vi "PQexecute.vi"(8 "error in":errorcluster, 10 "SQL querry":string, 11 "conn":u64) -> (0 "error out":errorcluster, 3 "conn_out":u64)   [LabVIEW 2019, in "libpqutility64.lvlib"]
uses:
  libpqutility64.lvlib
  libpqlv64/libpqlv64.lvlib
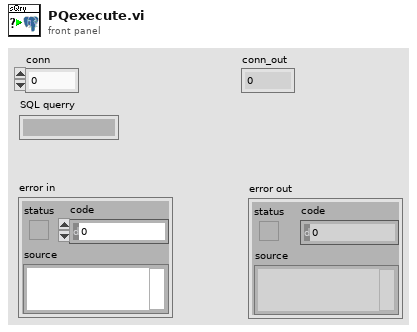
[diagram p1: front panel]
types:
  T1 = enum32{"PGRES_EMPTY_QUERY", "PGRES_COMMAND_OK", "PGRES_TUPLES_OK", "PGRES_COPY_OUT", "PGRES_COPY_IN", "PGRES_BAD_RESPONSE", "PGRES_NONFATAL_ERROR", "PGRES_FATAL_ERROR"}
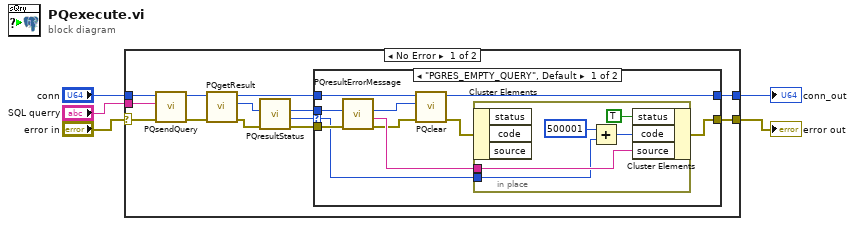
[diagram p0: block diagram]
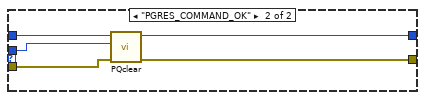
[diagram p2: hidden frame]
diagram:
  n1 = case shown="No Error" "error in" {
    selector: "error in" -> [w14 w39]
    tunnel: "conn" -> [w13 w40]
    tunnel: [w6 w40] -> w2
    tunnel: [w16 w39] -> w1
    tunnel: "SQL querry" -> [w15 _]
    frame No Error {
      n2 = call "PQsendQuery.vi"("error in (no error)"=w14, "query"=w15, "conn"=w13) -> ("error out"=w18:errorcluster, "conn_out"=w12:u64)  [unwired: 6 in, 1 out]
      n3 = call "PQgetResult.vi"("error in (no error)"=w18, "conn"=w12) -> ("error out"=w17:errorcluster, "PGresult"=w11:u64, "conn_out"=w7:u64)  [unwired: 7 in]
      n4 = call "PQresultStatus.vi"("error in (no error)"=w17, "res"=w11) -> ("error out"=w8:errorcluster, "PQresultStatus"=w10:T1, "res out"=w9:u64)  [unwired: 7 in]
      n5 = case shown="\"PGRES_EMPTY_QUERY\", Default" w10 {
        selector: w10 -> [w26 _]
        tunnel: [w25 w36] -> w16
        tunnel: w9 -> [w24 w38]
        tunnel: w8 -> [w28 w37]
        tunnel: w7 -> [w23 w35]
        tunnel: [w20 w34] -> w6
        frame "PGRES_EMPTY_QUERY", Default {
          n6 = call "PQresultErrorMessage.vi"("error in (no error)"=w28, "res"=w24) -> ("error out"=w22:errorcluster, "PQresultErrorMessage"=w27:string, "res out"=w21:u64)  [unwired: 7 in]
          n7 = call "PQclear.vi"("error in"=w22, "res"=w21, "conn"=w23) -> ("error out"=w19:errorcluster, "conn_out"=w20:u64)  [unwired: 7 in]
          n8 = in-place {
            in-place-border: w27 -> [w33]
            in-place-border: w26 -> [w30]
            n9 = in-place-cluster #1(w19) -> ()  [unwired: 3 out]
            n10 = Add(x=u32 500001, y=w30) -> (x+y=w29:u32)
            n11 = in-place-cluster #1("status"=TRUE, "code"=w29, "source"=w33) -> (w25:errorcluster)
          }
        }
        frame "PGRES_COMMAND_OK" {
          n12 = call "PQclear.vi"("error in"=w37, "res"=w38, "conn"=w35) -> ("error out"=w36:errorcluster, "conn_out"=w34:u64)  [unwired: 7 in]
        }
      }
    }
    frame Error {
    }
  }
  "conn_out" <- w2
  "error out" <- w1
